vi "Read BaseMeasures.vi"(8 "error in (no error)":errorcluster, 11 "AcPwrBase in":refnum<class "AcPwrBase.lvclass">) -> (0 "error out":errorcluster, 2 "BaseMeasures":T1[](array[typedef]), 3 "AcPwrBase out":refnum<class "AcPwrBase.lvclass">)   [LabVIEW 2014, in "AcPwrPlugins.lvlib" / "AcPwrBase.lvclass"]
uses:
  AcPwrBase.lvclass
  TypeDefs/BaseMeasure.ctl
  TypeDefs/MeasType.ctl
  AcPwrBase.lvclass/AcPwrBase.ctl
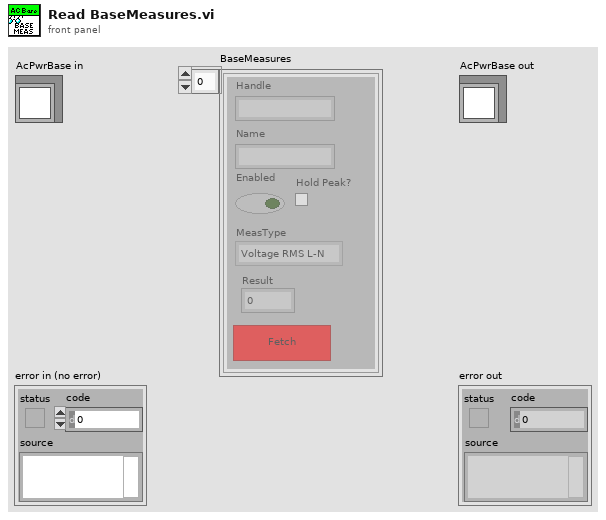
[diagram p1: front panel]
types:
  T1 = typedef "AcPwrPlugins.lvlib/AcPwrBase.lvclass/BaseMeasure.ctl" = cluster{"Handle":string, "Name":string, "Enabled":bool, "Result":dbl, "MeasType":T2, "btnMeasFetch":bool, "Hold Peak?":bool}
  T2 = typedef "AcPwrPlugins.lvlib/AcPwrBase.lvclass/MeasType.ctl" = enum16{"Voltage RMS L-N", "Current RMS", "Frequency", "Voltage DC", "Current DC", "Power Factor", "Current Peak", "Power VA", "Real Power", "Voltage THD", "Voltage EHD", "Voltage OHD", "Current THD", "Current EHD", "Current OHD", "Voltage RMS L-L", "Phase Angle", "Power DC", "Crest Factor"}
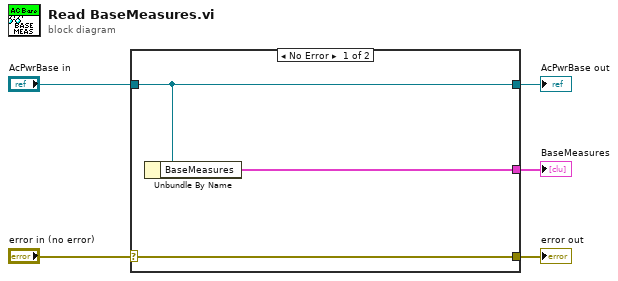
[diagram p0: block diagram]
diagram:
  n1 = case shown="No Error" "error in (no error)" {
    selector: "error in (no error)" -> [w8 w9]
    tunnel: [w8 w9] -> w4
    tunnel: [w7 w10] -> w2
    tunnel: "AcPwrBase in" -> [w7 w10]
    tunnel: [w6 _] -> w1
    frame No Error {
      n2 = Unbundle By Name(w7) -> ("BaseMeasures"=w6:T1[])
    }
    frame Error {
    }
  }
  "error out" <- w4
  "AcPwrBase out" <- w2
  "BaseMeasures" <- w1
